vi "FringeTrackerInputs.vi"(0 "SPEC":bool, 1 "WL":bool, 7 "error in (no error)":errorcluster) -> (4 "error out":errorcluster)   [LabVIEW 2009]
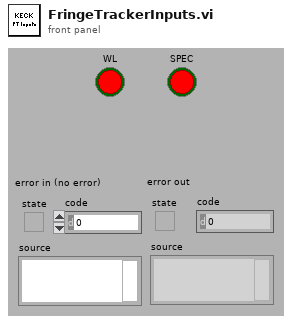
[diagram p1: front panel]
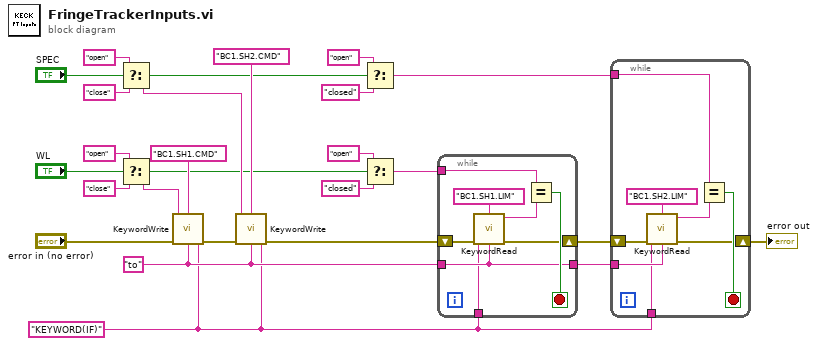
[diagram p0: block diagram]
diagram:
  w1 = "KEYWORD(IF)" ("Crate")
  w2 = "to"
  n1 = Select(t="open", s="SPEC", f="close") -> (s? t:f=w12:string)
  n2 = Select(t="open", s="WL", f="close") -> (s? t:f=w11:string)
  n3 = call "KeywordWrite.vi"("Crate"=w1, "Keyword"="BC1.SH1.CMD", "Value"=w11, "Service"=w2, "error in (no error)"="error in (no error)") -> ("error out"=w19:errorcluster)  [unwired: 4 out]
  n4 = call "KeywordWrite.vi"("Crate"=w1, "Keyword"="BC1.SH2.CMD", "Value"=w12, "Service"=w2, "error in (no error)"=w19) -> ("error out"=w16:errorcluster)  [unwired: 4 out]
  n5 = Select(t="open", s="SPEC", f="closed") -> (s? t:f=w3:string)
  n6 = Select(t="open", s="WL", f="closed") -> (s? t:f=w4:string)
  n7 = while {
    shift-right: [w29] -> w14
    shift-left: w16 -> [w32]
    tunnel: w2 -> [w27]
    tunnel: [w27] -> w13
    tunnel: w4 -> [w28]
    tunnel: w1 -> [w25]
    stop <- w30 stop-if-true
    n8 = call "KeywordRead.vi"("Keyword"="BC1.SH1.LIM", "Crate"=w25, "Service"=w27, "error in (no error)"=w32) -> ("Value"=w26:string, "error out"=w29:errorcluster)  [unwired: 1 in, 3 out]
    n9 = Equal?(x=w28, y=w26) -> (x = y?=w30:bool)
  }
  n10 = while {
    shift-right: [w37] -> w15
    shift-left: w14 -> [w40]
    tunnel: w13 -> [w35]
    tunnel: w3 -> [w36]
    tunnel: w1 -> [w33]
    stop <- w38 stop-if-true
    n11 = call "KeywordRead.vi"("Keyword"="BC1.SH2.LIM", "Crate"=w33, "Service"=w35, "error in (no error)"=w40) -> ("Value"=w34:string, "error out"=w37:errorcluster)  [unwired: 4 out]
    n12 = Equal?(x=w36, y=w34) -> (x = y?=w38:bool)
  }
  "error out" <- w15
